vi "Drive For Distance Controller.vi"(6 "Vision":bool, 8 "Command Iteration":i32, 9 "Speed":dbl, 10 "Distance (in)":dbl, 11 "RobotDriveDevRef":T1={"DevStatus"={"status"=FALSE, "code"=0, "source"=""}, "Motors[]"=[], "Square Inputs"=FALSE, "Max Output"=1.0}) -> (1 "Right Setpoint":dbl, 2 "Left Setpoint":dbl, 3 "Finished?":bool)   [LabVIEW 2016]
uses:
  <vilib>/Rock Robotics/WPI/RobotDrive/WPI_RobotDriveDevRef.ctl
  <vilib>/Rock Robotics/WPI/MotorControl/WPI_MotorControlDeviceRef.ctl
  <vilib>/Rock Robotics/WPI/MotorControl/WPI_MotorControlType.ctl
  <vilib>/Rock Robotics/SystemInterfaces/DIO/FPGA_DIOPWMChannel.ctl
  <vilib>/Rock Robotics/WPI/PWM/WPI_PWMDeadband.ctl
  Lidar/Lidar Global.vi
  NavX/NavX Global.vi
  <vilib>/Rock Robotics/Network Tables/NT Read Number.vi
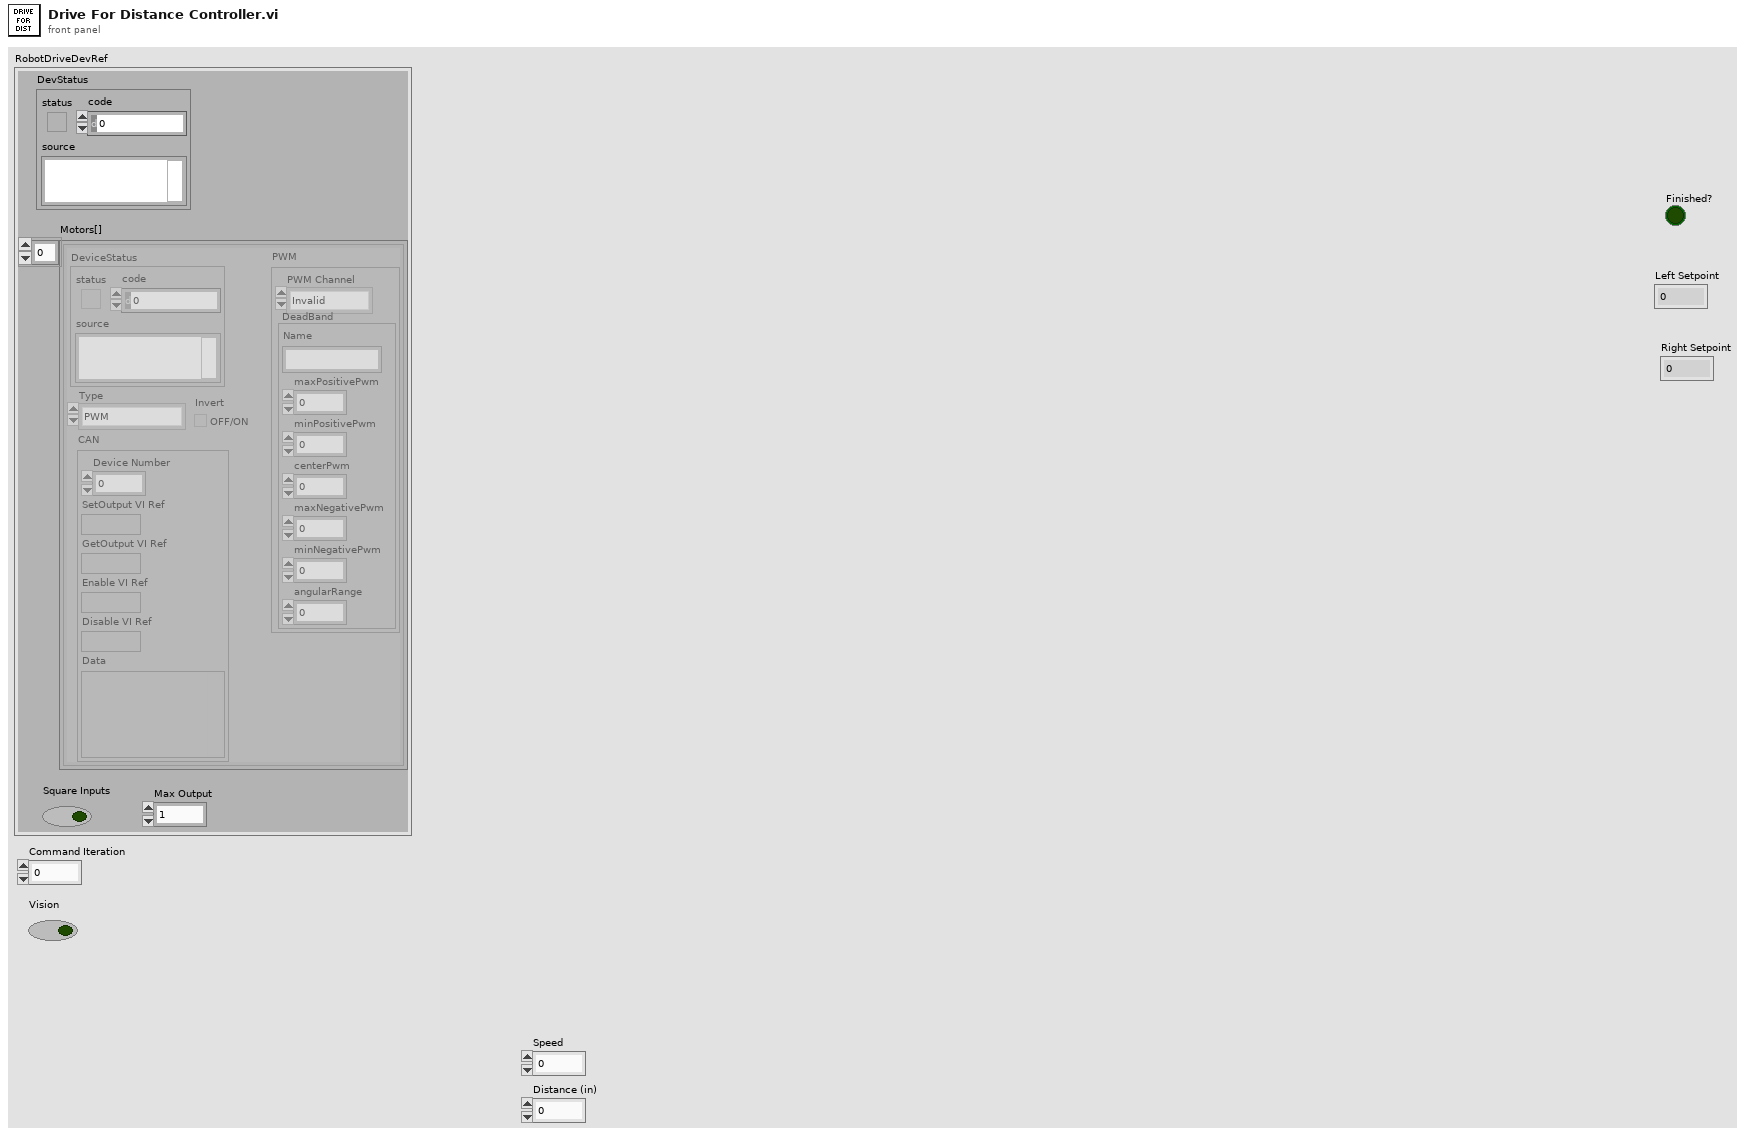
[diagram p1: front panel]
types:
  T1 = typedef "WPI_RobotDriveDevRef.ctl" = cluster{"DevStatus":errorcluster, "Motors[]":T2[], "Square Inputs":bool, "Max Output":dbl}
  T2 = typedef "WPI_MotorControlDeviceRef.ctl" = cluster{"DeviceStatus":errorcluster, "Type":T3, "PWM":cluster{"PWM Channel":T4, "DeadBand":T5}, "CAN":cluster{"Device Number":u8, "SetOutput VI Ref":variant, "GetOutput VI Ref":variant, "Enable VI Ref":variant, "Disable VI Ref":variant, "Data":variant}, "Invert":bool}
  T3 = typedef "WPI_MotorControlType.ctl" = enum16{"PWM", "CAN"}
  T4 = typedef "FPGA_DIOPWMChannel.ctl" = enum8{"PWM 0", "PWM 1", "PWM 2", "PWM 3", "PWM 4", "PWM 5", "PWM 6", "PWM 7", "PWM 8", "PWM 9", "PWM MXP 0", "PWM MXP 1", "PWM MXP 2", "PWM MXP 3", "PWM MXP 4", "PWM MXP 5", "PWM MXP 6", "PWM MXP 7", "PWM MXP 8", "PWM MXP 9", "Invalid"}
  T5 = typedef "WPI_PWMDeadband.ctl" = cluster{"Name":string, "maxPositivePwm":i32, "minPositivePwm":i32, "centerPwm":i32, "maxNegativePwm":i32, "minNegativePwm":i32, "angularRange":u16}
  T6 = cluster{"Yaw":dbl, "Roll":dbl, "Pitch":dbl, "Heading":dbl, "Fused Heading":dbl}
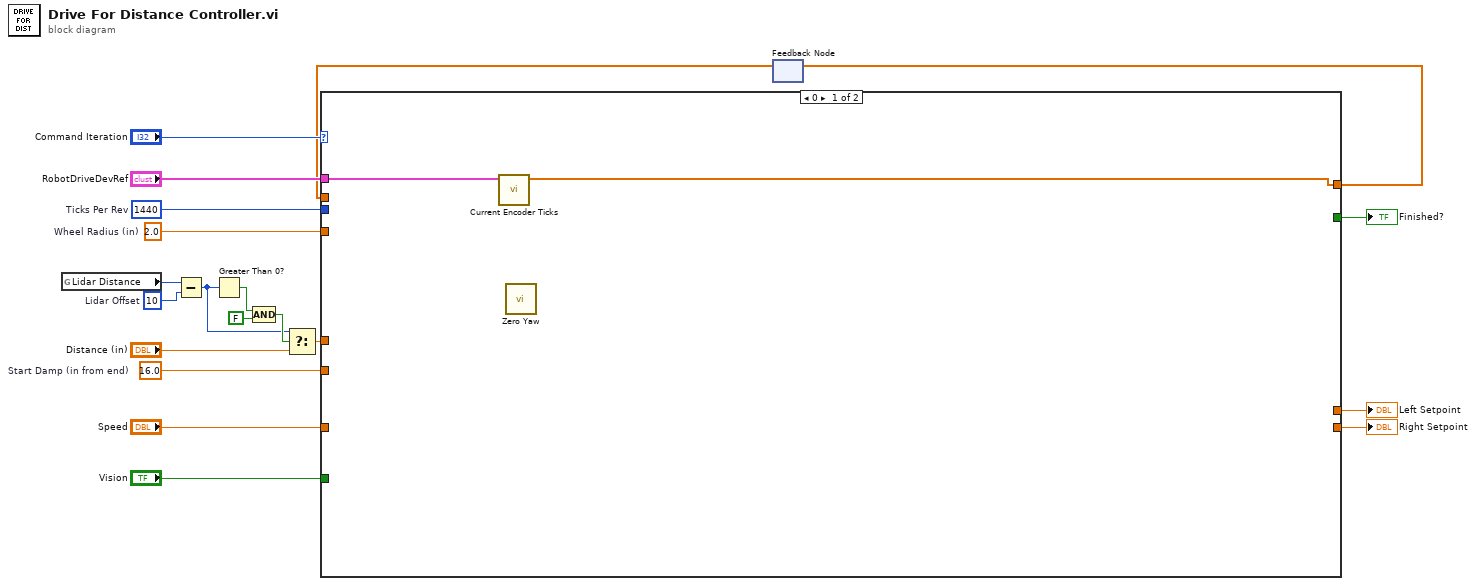
[diagram p0: block diagram]
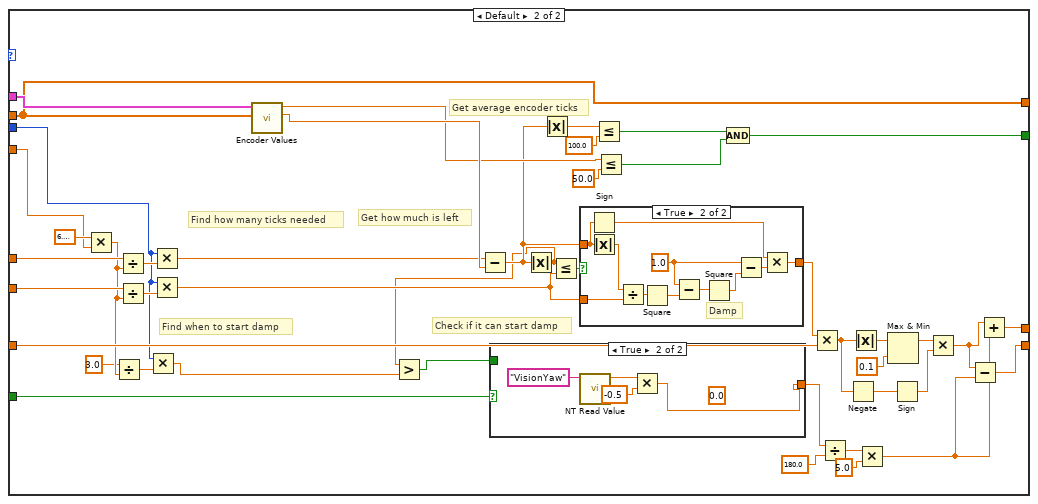
[diagram p2: hidden frame]
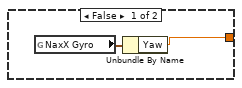
[diagram p3: hidden frame]
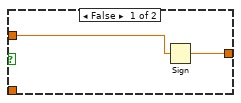
[diagram p4: hidden frame]
diagram:
  w2 = u16 10  # Lidar Offset
  w16 = 16.0  # Start Damp (in from end)
  w18 = 2.0  # Wheel Radius (in)
  w17 = 1440  # Ticks Per Rev
  n1 = global read "Lidar Global.vi" "Lidar Distance"() -> (w4:u16)
  n2 = Subtract(x=w4, y=w2) -> (x-y=w3:u16)
  n3 = Greater Than 0?(x=w3) -> (x > 0?=w5:bool)
  n4 = Compound Arithmetic op=AND(w5, FALSE ("value")) -> (w6:bool)
  n5 = Select(t=w3, s=w6, f="Distance (in)") -> (s? t:f=w8:dbl)
  n6 = feedback #1() -> (w10:dbl[])  [unwired: 1 in]
  n7 = case shown="0" "Command Iteration" {
    tunnel: "RobotDriveDevRef" -> [w22 w66]
    tunnel: w18 -> [_ w64]
    tunnel: w8 -> [_ w63]
    tunnel: w17 -> [_ w32]
    tunnel: w16 -> [_ w58]
    tunnel: [_ w46] -> w15
    tunnel: "Speed" -> [_ w59]
    tunnel: [_ w24] -> w13
    tunnel: [_ w26] -> w12
    tunnel: w10 -> [_ w37]
    tunnel: [w21 w37] -> w11
    tunnel: "Vision" -> [_ w36]
    frame 0 {
      n8 = call "Current Encoder Ticks.vi"("RobotDriveDevRef"=w22) -> ("Array"=w21:dbl[])  [unwired: 10 in]
      n9 = call <vilib>:"Zero Yaw.vi"() -> ()  [unwired: 12 in]
    }
    frame Default {
      # "Check if it can start damp"
      # "Get how much is left"
      # "Get average encoder ticks"
      # "Find how many ticks needed"
      # "Find when to start damp"
      n10 = Multiply(x=6.283185307179586, y=w64) -> (x*y=w31:dbl)
      n11 = Divide(x=3.0, y=w31) -> (x/y=w33:dbl)
      n12 = Divide(x=w63, y=w31) -> (x/y=w62:dbl)
      n13 = Divide(x=w58, y=w31) -> (x/y=w57:dbl)
      n14 = Multiply(x=w32, y=w33) -> (x*y=w29:dbl)
      n15 = Multiply(x=w32, y=w62) -> (x*y=w54:dbl)
      n16 = Multiply(x=w32, y=w57) -> (x*y=w47:dbl)
      n17 = call "Encoder Values.vi"("Array"=w37, "RobotDriveDevRef"=w66) -> ("Position"=w55:dbl, "Velocity"=w42:dbl)  [unwired: 8 in]
      n18 = Subtract(x=w54, y=w55) -> (x-y=w34:dbl)
      n19 = Absolute Value(x=w34) -> (abs(x)=w27:dbl)
      n20 = Greater?(x=w27, y=w29) -> (0:w28:bool)
      n21 = case shown="True" w36 {
        tunnel: [w67 w69] -> w35
        tunnel: w28 -> [_ _]
        frame False {
          n22 = global read "NavX Global.vi" "NaxX Gyro"() -> (w68:T6)
          n23 = Unbundle By Name(w68) -> ("Yaw"=w67:dbl)
        }
        frame True {
          (unwired) 0.0 ("f")
          n24 = call-poly <vilib>:"NT Read Value.vi"("Name"="VisionYaw") -> ("Numeric"=w70:dbl)  [unwired: 9 in, 1 out]
          n25 = Multiply(x=w70, y=-0.5) -> (x*y=w69:dbl)
        }
      }
      n26 = Absolute Value(x=w34) -> (abs(x)=w48:dbl)
      n27 = Less Or Equal?(x=w27, y=w47) -> (x <= y?=w61:bool)
      n28 = case shown="True" w61 {
        tunnel: w34 -> [w73 w78]
        tunnel: w47 -> [_ w81]
        tunnel: [w74 w76] -> w60
        frame False {
          n29 = Sign(1:w73) -> (0:w74:dbl)
        }
        frame True {
          w83 = 1.0
          # "Damp"
          n30 = Sign(1:w78) -> (0:w75:dbl)
          n31 = Absolute Value(x=w78) -> (abs(x)=w79:dbl)
          n32 = Divide(x=w79, y=w81) -> (x/y=w80:dbl)
          n33 = Square(x=w80) -> (x^2=w85:dbl)
          n34 = Subtract(x=w83, y=w85) -> (x-y=w84:dbl)
          n35 = Square(x=w84) -> (x^2=w82:dbl)
          n36 = Subtract(x=w83, y=w82) -> (x-y=w77:dbl)
          n37 = Multiply(x=w75, y=w77) -> (x*y=w76:dbl)
        }
      }
      n38 = Less Or Equal?(x=w48, y=100.0) -> (x <= y?=w44:bool)
      n39 = Less Or Equal?(x=w42, y=50.0) -> (x <= y?=w43:bool)
      n40 = Compound Arithmetic op=AND(w44, w43) -> (w46:bool)
      n41 = Multiply(x=w60, y=w59) -> (x*y=w51:dbl)
      n42 = Divide(x=w35, y=180.0) -> (x/y=w40:dbl)
      n43 = Negate(x=w51) -> (-x=w50:dbl)
      n44 = Absolute Value(x=w51) -> (abs(x)=w52:dbl)
      n45 = Multiply(x=w40, y=5.0) -> (x*y=w23:dbl)
      n46 = Max & Min(x=w52, y=0.1) -> (max(x,y)=w49:dbl)  [unwired: 1 out]
      n47 = Sign(1:w50) -> (0:w38:dbl)
      n48 = Multiply(x=w49, y=w38) -> (x*y=w25:dbl)
      n49 = Subtract(x=w25, y=w23) -> (x-y=w24:dbl)
      n50 = Add(x=w25, y=w23) -> (x+y=w26:dbl)
    }
  }
  "Finished?" <- w15
  "Left Setpoint" <- w12
  "Right Setpoint" <- w13
  n51 = feedback-in #1(w11) -> ()
